vi "一致性结果转换.vi"(11 "一致性结果字符串":string="111111111100000011") -> (3 "数字":u16)   [LabVIEW 2017]
panel:
  out "数字 3":u32
  out "无符号字节数组":u8[](array[numeric])
  out "数组 3":bool[](array[boolean])
  out "数组 2":string[](array[string])
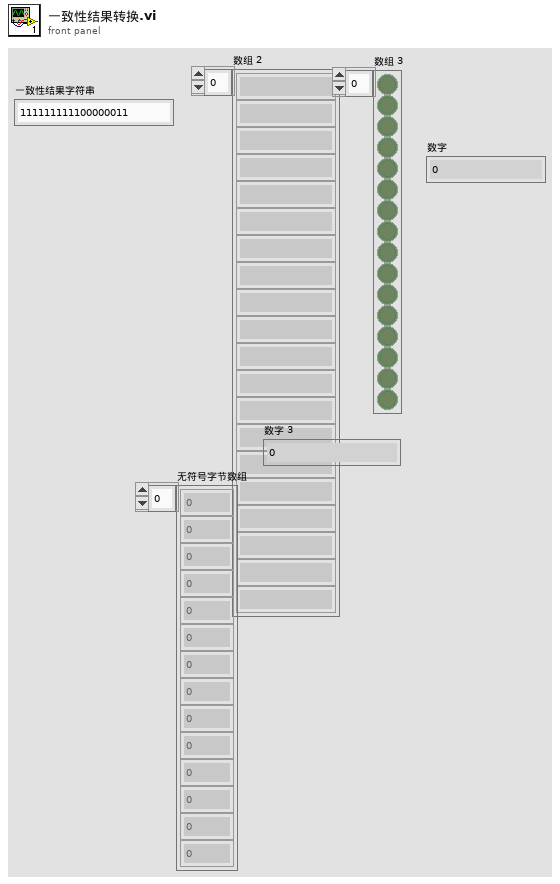
[diagram p1: front panel]
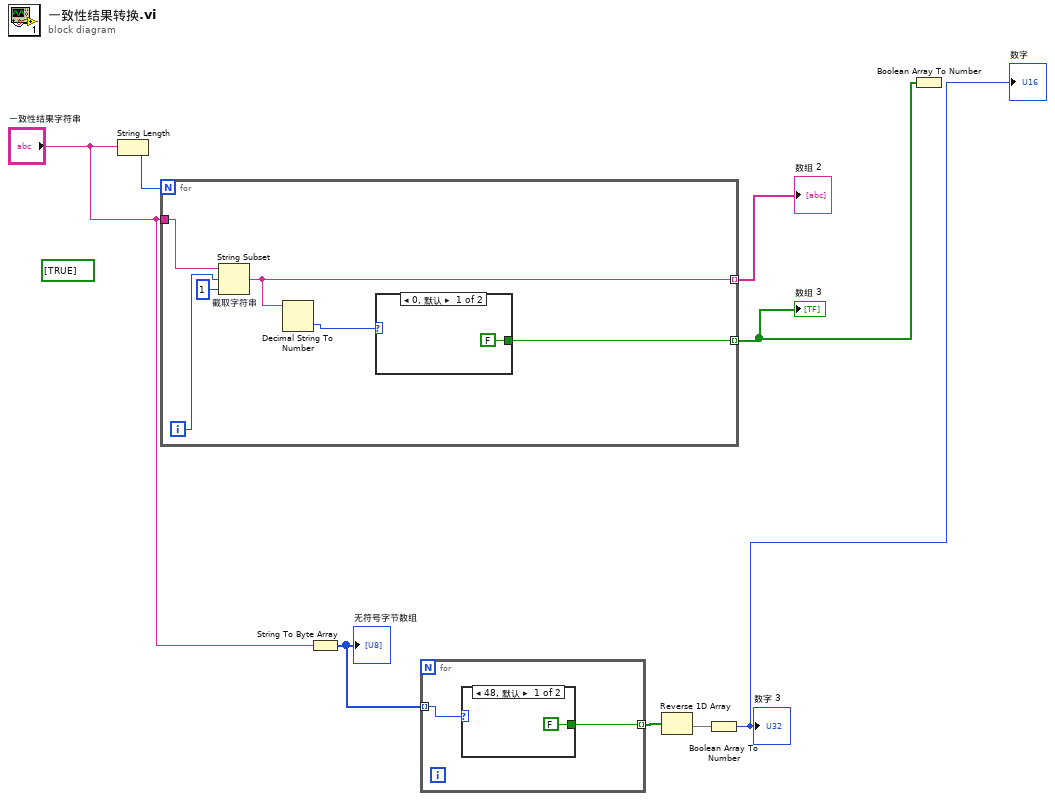
[diagram p0: block diagram]
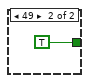
[diagram p2: hidden frame]
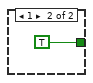
[diagram p3: hidden frame]
diagram:
  (unwired) bool[] [TRUE]
  n1 = String Length(string="一致性结果字符串") -> (length=w8:i32)
  n2 = for {
    N: w8 -> [_]
    tunnel: "一致性结果字符串" -> [w14]
    tunnel: [w11] -> w7 mode=indexing
    tunnel: [w9] -> w6 mode=indexing
    i -> [w12]
    n3 = String Subset "截取字符串"(string=w14, offset (0)=w12, length (rest)=1 ("长度（剩余）")) -> (substring=w11:string)
    n4 = Decimal String To Number(string=w11) -> (number=w10:i32)  [unwired: 2 in, 1 out]
    n5 = case shown="0, 默认" w10 {
      tunnel: [FALSE TRUE] -> w9
      frame 0, Default {
      }
      frame 1 {
      }
    }
  }
  "数组 2" <- w7
  "数组 3" <- w6
  n6 = String To Byte Array(string="一致性结果字符串") -> (unsigned byte array=w5:u8[])
  "无符号字节数组" <- w5
  n7 = for {
    tunnel: w5 -> [w18] mode=indexing
    tunnel: [w17] -> w4 mode=indexing
    n8 = case shown="48, 默认" w18 {
      tunnel: [FALSE TRUE] -> w17
      frame 48, Default {
      }
      frame 49 {
      }
    }
  }
  n9 = Reverse 1D Array(array=w4) -> (reversed array=w3:bool[])
  n10 = Boolean Array To Number(Boolean array=w3) -> (number=→"数字" →"数字 3":u32)
  n11 = Boolean Array To Number(Boolean array=w6) -> ()  [unwired: 1 out]
